vi "Logger.vi"(0 "Record":refnum<vi>, 1 "Indicators":T6, 2 "Time Stamp":refnum<vi>, 5 "Exit":refnum<vi>, 7 "Visual Data":T1, 9 "Period [ms]":i32=50, 11 "error in (no error)":errorcluster, 12 "File Path Control":refnum<vi>, 13 "Configuration":T5, 14 "Filename":string="RITA") -> (15 "error out":errorcluster)   [LabVIEW 2012, in "Logger VIs.lvlib"]
uses:
  Logger VIs.lvlib
  State.ctl
  <vilib>/silver_ctls/ArrayMatrixCluster/Real Matrix NI_Silver.ctl
  <vilib>/vision/Image Controls.llb/IMAQ Image.ctl
  <vilib>/Utility/xml.llb/Write to XML File(string).vi
panel:
  out "Transformation":T3
  out "Calibration":T4
  out "Angles":cluster{"Azimut":dbl, "Elevation":dbl}
  out "Surface Space":dbl
  out "ms from start":dbl
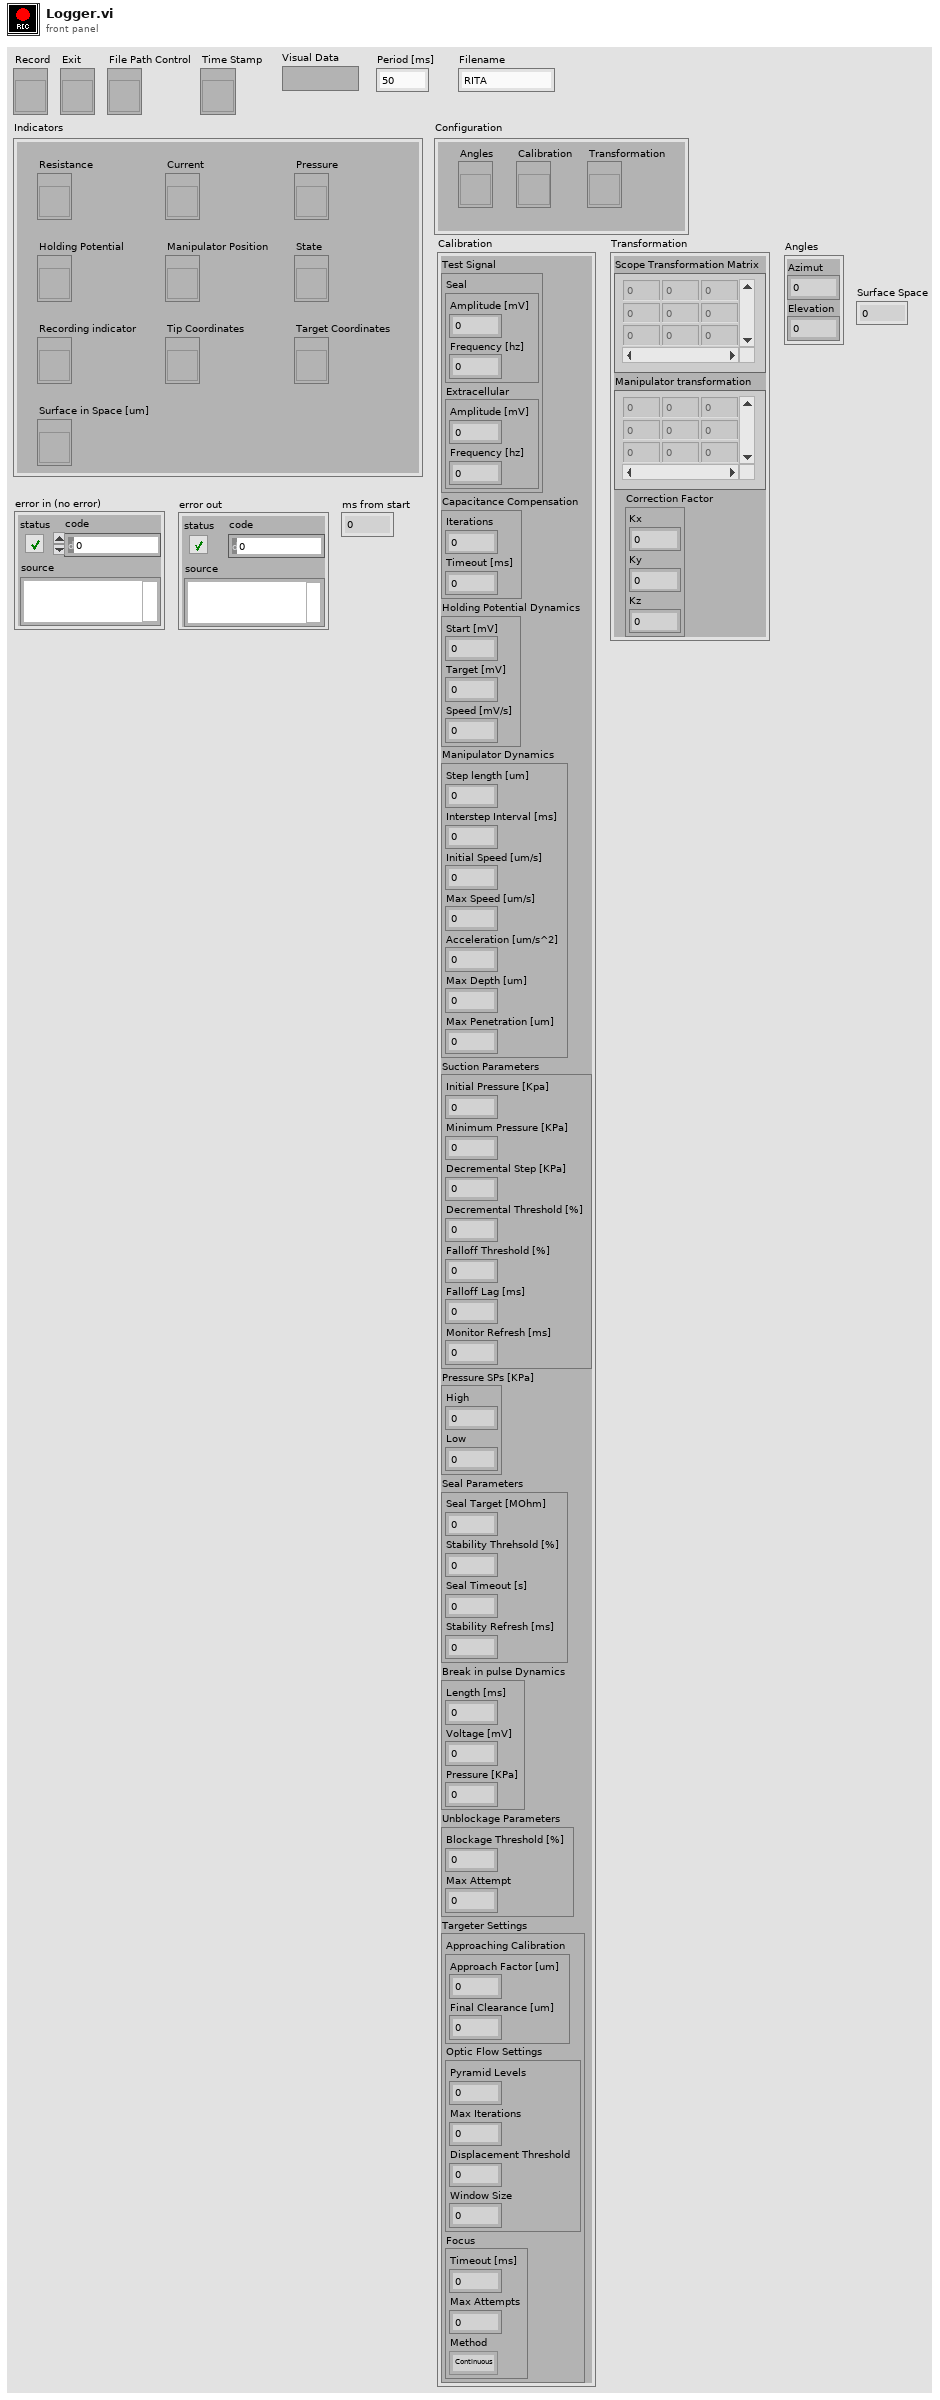
[diagram p1: front panel]
types:
  T1 = typedef "IMAQ Image.ctl" = refnum<image>
  T2 = typedef "Real Matrix NI_Silver.ctl" = dbl[][]
  T3 = cluster{"Scope Transformation Matrix":T2, "Manipulator transformation":T2, "Correction Factor":cluster{"Kx":dbl, "Ky":dbl, "Kz":dbl}}
  T4 = cluster{"Test Signal":cluster{"Seal":cluster{"Amplitude [mV]":i32, "Frequency [hz]":u16}, "Extracellular":cluster{"Amplitude [mV]":i32, "Frequency [hz]":u16}}, "Capacitance Compensation":cluster{"Iterations":i32, "Timeout [ms]":u32}, "Holding Potential Dynamics":cluster{"Start [mV]":dbl, "Target [mV]":dbl, "Speed [mV/s]":dbl}, "Manipulator Dynamics":cluster{"Step length [um]":dbl, "Interstep Interval [ms]":u32, "Initial Speed [um/s]":dbl, "Max Speed [um/s]":dbl, "Acceleration [um/s^2]":dbl, "Max Depth [um]":dbl, "Max Penetration [um]":dbl}, "Suction Parameters":cluster{"Initial Pressure [Kpa]":dbl, "Minimum Pressure [KPa]":dbl, "Decremental Step [KPa]":dbl, "Decremental Threshold [%]":dbl, "Falloff Threshold [%]":dbl, "Falloff Lag [ms]":dbl, "Monitor Refresh [ms]":dbl}, "Pressure SPs [KPa]":cluster{"High":dbl, "Low":dbl}, "Seal Parameters":cluster{"Seal Target [MOhm]":dbl, "Stability Threhsold [%]":dbl, "Seal Timeout [s]":dbl, "Stability Refresh [ms]":dbl}, "Break in pulse Dynamics":cluster{"Length [ms]":dbl, "Voltage [mV]":dbl, "Pressure [KPa]":dbl}, "Unblockage Parameters":cluster{"Blockage Threshold [%]":dbl, "Max Attempt":i32}, "Targeter Settings":cluster{"Approaching Calibration":cluster{"Approach Factor [um]":dbl, "Final Clearance [um]":dbl}, "Optic Flow Settings":cluster{"Pyramid Levels":i32, "Max Iterations":i32, "Displacement Threshold":dbl, "Window Size":i32}, "Focus":cluster{"Timeout [ms]":u32, "Max Attempts":u32, "Method":enum16{"Continuous", "On Demand"}}}}
  T5 = cluster{"Angles":refnum<vi>, "Calibration":refnum<vi>, "Transformation":refnum<vi>}
  T6 = cluster{"Current":refnum<vi>, "Holding Potential":refnum<vi>, "Recording indicator":refnum<vi>, "Pressure":refnum<vi>, "Resistance":refnum<vi>, "Manipulator Position":refnum<vi>, "Tip Coordinates":refnum<vi>, "Target Coordinates":refnum<vi>, "Surface in Space [um]":refnum<vi>, "State":refnum<vi>}
  T7 = enum16{"open", "replace", "create", "open or create", "replace or create", "replace or create with confirmation"}
  T8 = cluster{"Value":dbl, "Value 2":dbl, "Value 3":dbl}
  T9 = cluster{"X [um]":dbl, "Y [um]":dbl, "Z [um]":dbl}
  T10 = typedef "State.ctl" = enum16{"READY", "LOAD", "LOCALIZATION", "HUNTING", "SEAL", "BREAKIN", "WCR", "ALIGN", "APPROACH", "TARGETING"}
  T11 = cluster{"Scope Transformation Matrix":T2, "Manipulator transformation":T2, "Coorection Factor":cluster{"Kx":dbl, "Ky":dbl, "Kz":dbl}}
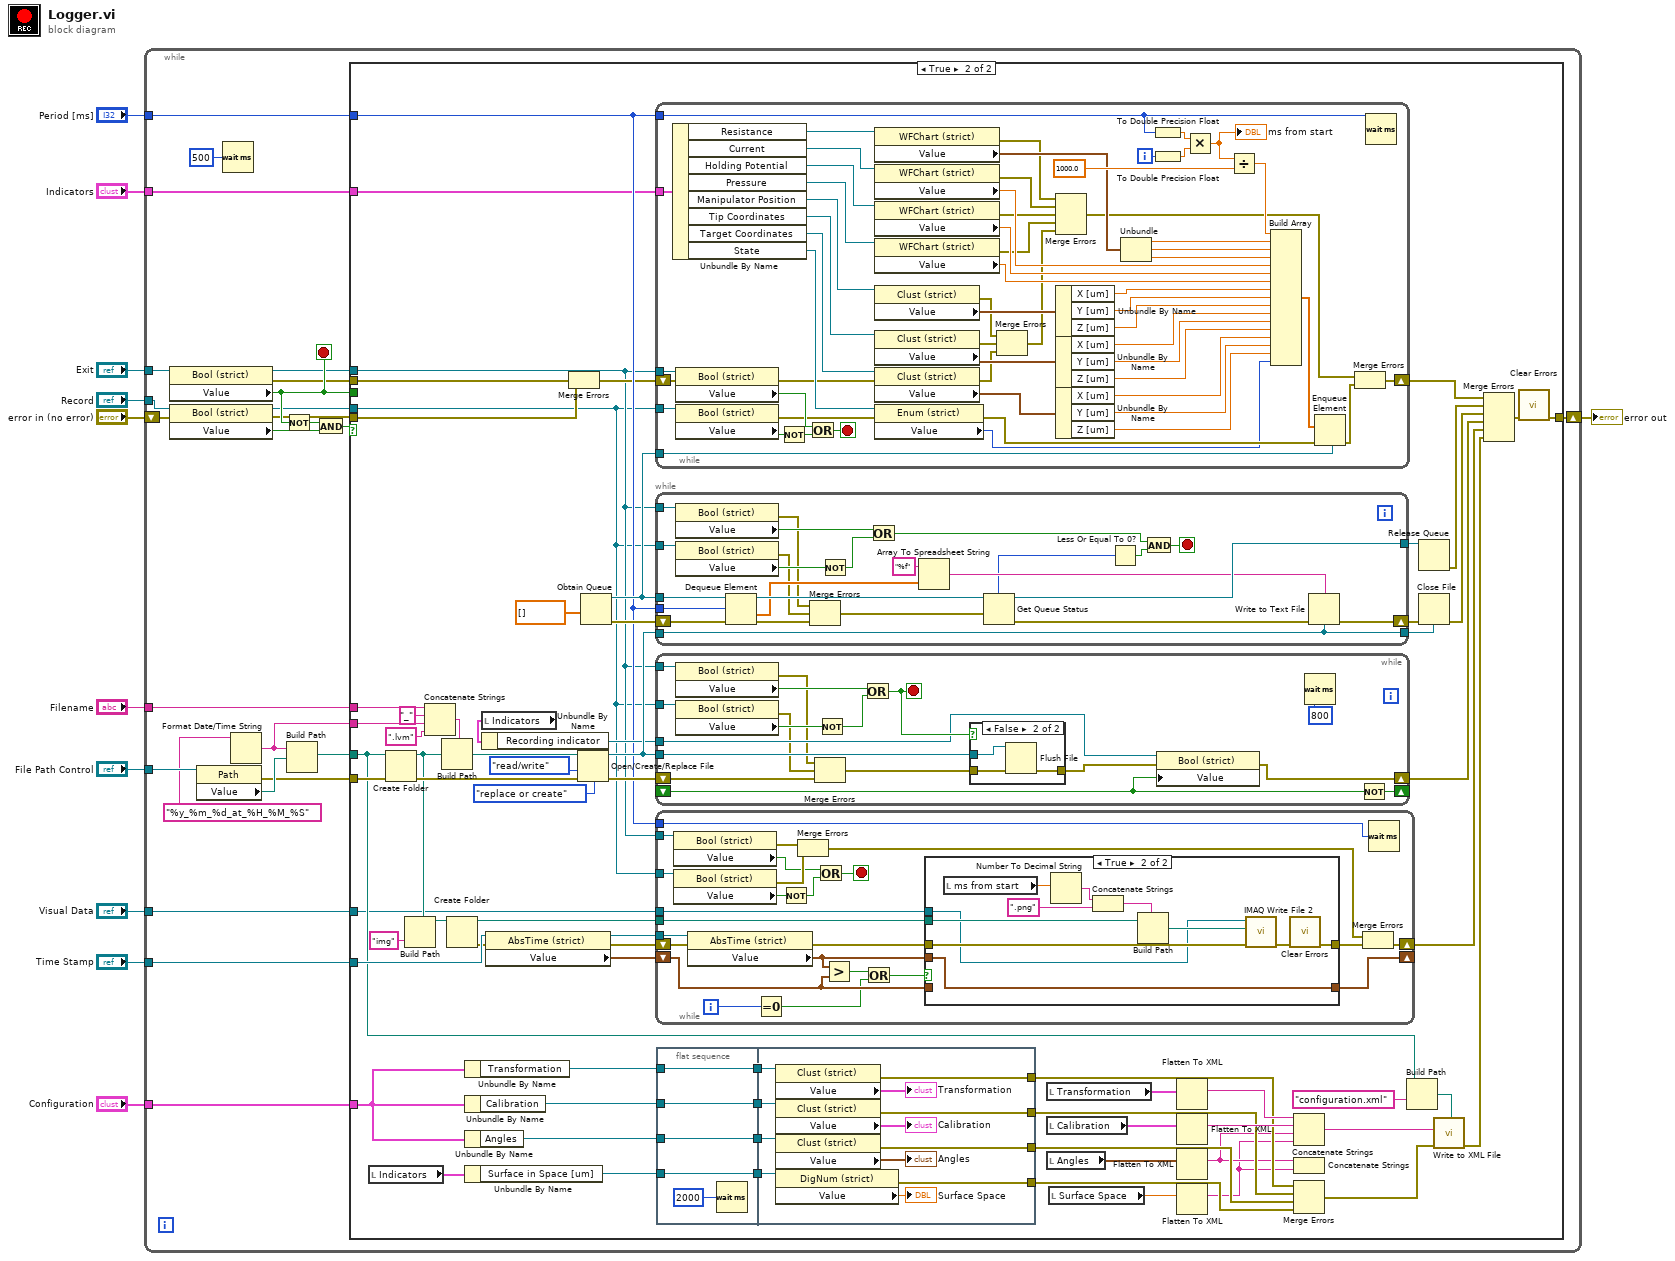
[diagram p0: block diagram]
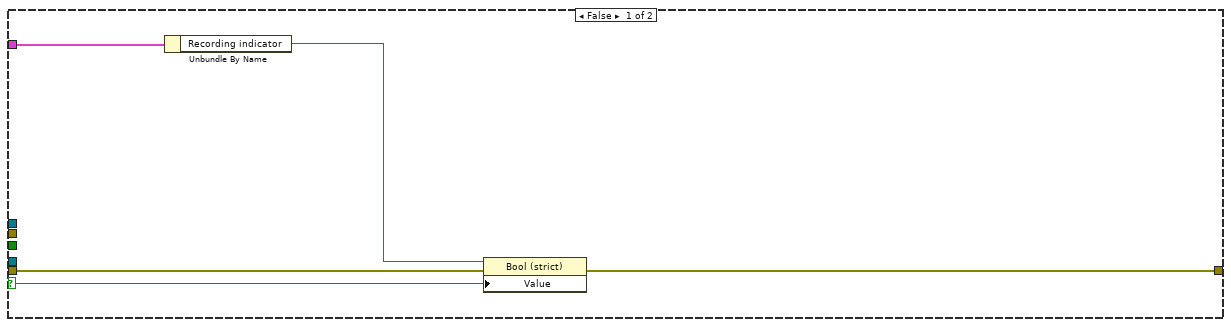
[diagram p2: hidden frame]
diagram:
  n1 = while {
    tunnel: "Indicators" -> [w35]
    tunnel: "Period [ms]" -> [w36]
    tunnel: "Exit" -> [w16]
    tunnel: "Record" -> [w17]
    shift-right: [w31] -> w7
    shift-left: "error in (no error)" -> [w13]
    tunnel: "File Path Control" -> [w32]
    tunnel: "Filename" -> [w30]
    tunnel: "Time Stamp" -> [w15]
    tunnel: "Configuration" -> [w14]
    tunnel: "Visual Data" -> [w12]
    stop <- w33 stop-if-true
    n2 = property class="Bool (strict)"(reference=w16) -> (reference out=w28:refnum<vi>, error out=w20:errorcluster, "Value"=w33:bool)  [unwired: 1 in]
    n3 = property class="Bool (strict)"(reference=w17, error in=w13) -> (reference out=w29:refnum<vi>, error out=w19:errorcluster, "Value"=w26:bool)
    n4 = property class="Path"(reference=w32) -> (error out=w21:errorcluster, "Value"=w24:path)  [unwired: 1 in, 1 out]
    n5 = Wait (ms)(milliseconds to wait=u32 500) -> ()  [unwired: 1 out]
    n6 = Format Date/Time String(time format string (%c)="%y_%m_%d_at_%H_%M_%S") -> (date/time string=w22:string)  [unwired: 2 in]
    n7 = Not(x=w33) -> (.not. x?=w25:bool)
    n8 = Build Path(base path=w24, name or relative path=w22) -> (appended path=w23:path)
    n9 = And(x=w25, y=w26) -> (x .and. y?=w27:bool)
    n10 = case shown="True" w27 {
      selector: w27 -> [w39 _]
      tunnel: w35 -> [w41 w79]
      tunnel: w36 -> [_ w80]
      tunnel: w29 -> [_ w48]
      tunnel: w33 -> [_ _]
      tunnel: w28 -> [_ w49]
      tunnel: [w38 w44] -> w31
      tunnel: w23 -> [_ w71]
      tunnel: w22 -> [_ w96]
      tunnel: w30 -> [_ w90]
      tunnel: w21 -> [_ w92]
      tunnel: w20 -> [_ w51]
      tunnel: w19 -> [w37 w50]
      tunnel: w15 -> [_ w85]
      tunnel: w14 -> [_ w73]
      tunnel: w12 -> [_ w46]
      frame False {
        n11 = Unbundle By Name(w41) -> ("Recording indicator"=w40:refnum<vi>)
        n12 = property class="Bool (strict)"(reference=w40, error in=w37, "Value"=w39) -> (error out=w38:errorcluster)  [unwired: 1 out]
      }
      frame True {
        n13 = local read "Indicators"() -> (w69:T6)
        n14 = Create Folder(path (use dialog)=w71, error in=w92) -> (created path=w93:path, error out=w94:errorcluster)  [unwired: 1 in, 1 out]
        n15 = Build Path(base path=w93, name or relative path="img") -> (appended path=w88:path)
        n16 = Concatenate Strings(w90, "_" ("string"), w96, ".lvm" ("time format string (%c)")) -> (w97:string)
        n17 = Build Path(base path=w93, name or relative path=w97) -> (appended path=w95:path)
        n18 = Create Folder(path (use dialog)=w88) -> (created path=w86:path, error out=w84:errorcluster)  [unwired: 2 in, 1 out]
        n19 = Unbundle By Name(w73) -> ("Transformation"=w76:refnum<vi>)
        n20 = Unbundle By Name(w73) -> ("Calibration"=w74:refnum<vi>)
        n21 = Unbundle By Name(w73) -> ("Angles"=w72:refnum<vi>)
        n22 = Unbundle By Name(w69) -> ("Surface in Space [um]"=w43:refnum<vi>)
        n23 = local read "Indicators"() -> (w75:T6)
        n24 = Unbundle By Name(w75) -> ("Recording indicator"=w103:refnum<vi>)
        n25 = property class="AbsTime (strict)"(reference=w85, error in=w84) -> (reference out=w81:refnum<vi>, error out=w82:errorcluster, "Value"=w83:timestamp)
        n26 = Merge Errors(w51, w50) -> (w52:errorcluster)
        n27 = Open/Create/Replace File(file path (use dialog)=w95, error in=w94, operation (0:open)=T7."replace or create", access (0:read/write)=enum16{"read/write", "read-only", "write-only"}."read/write") -> (refnum out=w107:refnum<file>, error out=w108:errorcluster)  [unwired: 2 in, 1 out]
        n28 = Obtain Queue(element data type=dbl[] [] ("array")) -> (queue out=w109:refnum<queue>, error out=w105:errorcluster)  [unwired: 4 in, 1 out]
        n29 = while {
          tunnel: w109 -> [w226]
          tunnel: w79 -> [w223]
          tunnel: w49 -> [w207]
          tunnel: w48 -> [w206]
          tunnel: w80 -> [w198]
          shift-right: [w180] -> w102
          shift-left: w52 -> [w168]
          i -> [w199]
          stop <- w205 stop-if-true
          n30 = Unbundle By Name(w223) -> ("Resistance"=w222:refnum<vi>, "Current"=w221:refnum<vi>, "Holding Potential"=w219:refnum<vi>, "Pressure"=w216:refnum<vi>, "Manipulator Position"=w215:refnum<vi>, "Tip Coordinates"=w194:refnum<vi>, "Target Coordinates"=w193:refnum<vi>, "State"=w196:refnum<vi>)
          n31 = property class="Bool (strict)"(reference=w207, error in=w168) -> (error out=w191:errorcluster, "Value"=w208:bool)  [unwired: 1 out]
          n32 = property class="Bool (strict)"(reference=w206) -> (error out=w190:errorcluster, "Value"=w209:bool)  [unwired: 1 in, 1 out]
          n33 = Not(x=w209) -> (.not. x?=w210:bool)
          n34 = Or(x=w208, y=w210) -> (x .or. y?=w205:bool)
          n35 = property class="WFChart (strict)"(reference=w222) -> (error out=w185:errorcluster, "Value"=w203:T8)  [unwired: 1 in, 1 out]
          n36 = property class="WFChart (strict)"(reference=w221) -> (error out=w186:errorcluster, "Value"=w220:dbl)  [unwired: 1 in, 1 out]
          n37 = property class="WFChart (strict)"(reference=w219) -> (error out=w187:errorcluster, "Value"=w218:dbl)  [unwired: 1 in, 1 out]
          n38 = property class="WFChart (strict)"(reference=w216) -> (error out=w188:errorcluster, "Value"=w217:dbl)  [unwired: 1 in, 1 out]
          n39 = property class="Clust (strict)"(reference=w215) -> (error out=w182:errorcluster, "Value"=w214:T9)  [unwired: 1 in, 1 out]
          n40 = property class="Clust (strict)"(reference=w194) -> (error out=w183:errorcluster, "Value"=w195:T9)  [unwired: 1 in, 1 out]
          n41 = property class="Clust (strict)"(reference=w193, error in=w191) -> (error out=w184:errorcluster, "Value"=w192:T9)  [unwired: 1 out]
          n42 = property class="Enum (strict)"(reference=w196, error in=w190) -> (error out=w189:errorcluster, "Value"=w177:T10)  [unwired: 1 out]
          n43 = Merge Errors(w182, w183, w184) -> (w181:errorcluster)
          n44 = Merge Errors(w185, w186, w187, w188, w181) -> (w179:errorcluster)
          n45 = Unbundle By Name(w214) -> ("X [um]"=w213:dbl, "Y [um]"=w212:dbl, "Z [um]"=w211:dbl)
          n46 = Unbundle By Name(w195) -> ("X [um]"=w174:dbl, "Y [um]"=w173:dbl, "Z [um]"=w172:dbl)
          n47 = Unbundle By Name(w192) -> ("X [um]"=w171:dbl, "Y [um]"=w170:dbl, "Z [um]"=w169:dbl)
          n48 = Unbundle(w203) -> ("Value"=w202:dbl, "Value 2"=w201:dbl, "Value 3"=w200:dbl)
          n49 = To Double Precision Float(number=w198) -> (double precision float=w176:dbl)
          n50 = To Double Precision Float(number=w199) -> (double precision float=w175:dbl)
          n51 = Multiply(x=w176, y=w175) -> (x*y=w197:dbl)
          "ms from start" <- w197
          n52 = Divide(x=w197, y=1000.0) -> (x/y=w204:dbl)
          n53 = Build Array(w204, w202, w201, w200, w220, w218, w217, w213, w212, w211, w174, w173, w172, w171, w170, w169, w177) -> (w224:dbl[])
          n54 = Enqueue Element(queue=w226, element=w224, error in (no error)=w189) -> (error out=w178:errorcluster)  [unwired: 1 in, 2 out]
          n55 = Merge Errors(w179, w178) -> (w180:errorcluster)
          n56 = Wait (ms)(milliseconds to wait=w198) -> ()  [unwired: 1 out]
        }
        n57 = while {
          tunnel: [w249] -> w113
          tunnel: w109 -> [w248]
          tunnel: w49 -> [w246]
          tunnel: w48 -> [w245]
          tunnel: w107 -> [w236]
          tunnel: [w236] -> w106
          tunnel: w80 -> [w231]
          shift-right: [w247] -> w104
          shift-left: w105 -> [w232]
          stop <- w237 stop-if-true
          n58 = property class="Bool (strict)"(reference=w246) -> (error out=w228:errorcluster, "Value"=w240:bool)  [unwired: 1 in, 1 out]
          n59 = property class="Bool (strict)"(reference=w245) -> (error out=w229:errorcluster, "Value"=w239:bool)  [unwired: 1 in, 1 out]
          n60 = Dequeue Element(queue=w248, timeout in ms (-1)=w231, error in (no error)=w232) -> (element=w243:dbl[], error out=w230:errorcluster)  [unwired: 2 out]
          n61 = Merge Errors(w228, w229, w230) -> (w227:errorcluster)
          n62 = Not(x=w239) -> (.not. x?=w241:bool)
          n63 = Or(x=w240, y=w241) -> (x .or. y?=w238:bool)
          n64 = Array To Spreadsheet String(array=w243, 3:"%f" ("format string")) -> (spreadsheet string=w244:string)  [unwired: 1 out]
          n65 = Get Queue Status(queue=w248, error in (no error)=w227) -> (queue out=w249:refnum<queue>, error out=w242:errorcluster, # elements in queue=w234:i32)  [unwired: 6 out]
          n66 = Less Or Equal To 0?(x=w234) -> (x <= 0?=w233:bool)
          n67 = And(x=w238, y=w233) -> (x .and. y?=w237:bool)
          n68 = Write to Text File(file (use dialog)=w236, text=w244, error in=w242) -> (error out=w247:errorcluster)  [unwired: 1 in, 2 out]
        }
        n69 = while {
          tunnel: w107 -> [w266]
          tunnel: w49 -> [w264]
          tunnel: w48 -> [w263]
          shift-right: [w256] -> w99
          shift-left: w108 -> [w251]
          shift-right: [w259] -> _
          shift-left: _ -> [w258]
          tunnel: w103 -> [w254]
          stop <- w257 stop-if-true
          n70 = property class="Bool (strict)"(reference=w264) -> (error out=w253:errorcluster, "Value"=w261:bool)  [unwired: 1 in, 1 out]
          n71 = property class="Bool (strict)"(reference=w263) -> (error out=w252:errorcluster, "Value"=w262:bool)  [unwired: 1 in, 1 out]
          n72 = Merge Errors(w253, w252, w251) -> (w250:errorcluster)
          n73 = Not(x=w262) -> (.not. x?=w260:bool)
          n74 = Or(x=w261, y=w260) -> (x .or. y?=w257:bool)
          n75 = case shown="False" w257 {
            tunnel: w266 -> [_ w270]
            tunnel: w250 -> [w267 w269]
            tunnel: [w267 w268] -> w255
            frame True {
            }
            frame False {
              n76 = Flush File(refnum=w270, error in=w269) -> (error out=w268:errorcluster)  [unwired: 1 out]
            }
          }
          n77 = property class="Bool (strict)"(reference=w254, error in=w255, "Value"=w258) -> (error out=w256:errorcluster)  [unwired: 1 out]
          n78 = Wait (ms)(milliseconds to wait=u32 800) -> ()  [unwired: 1 out]
          n79 = Not(x=w258) -> (.not. x?=w259:bool)
        }
        n80 = while {
          tunnel: w86 -> [w154]
          shift-right: [w139] -> w98
          shift-left: w82 -> [w147]
          shift-right: [w143] -> _
          shift-left: w83 -> [w144]
          tunnel: w81 -> [w148]
          tunnel: w49 -> [w142]
          tunnel: w48 -> [w141]
          tunnel: w80 -> [w136]
          tunnel: w46 -> [w135]
          i -> [w134]
          stop <- w151 stop-if-true
          n81 = property class="Bool (strict)"(reference=w142) -> (error out=w149:errorcluster, "Value"=w137:bool)  [unwired: 1 in, 1 out]
          n82 = property class="Bool (strict)"(reference=w141) -> (error out=w150:errorcluster, "Value"=w153:bool)  [unwired: 1 in, 1 out]
          n83 = property class="AbsTime (strict)"(reference=w148, error in=w147) -> (error out=w146:errorcluster, "Value"=w145:timestamp)  [unwired: 1 out]
          n84 = Equal To 0?(x=w134) -> (x = 0?=w131:bool)
          n85 = Not(x=w153) -> (.not. x?=w152:bool)
          n86 = Merge Errors(w149, w150) -> (w138:errorcluster)
          n87 = Or(x=w137, y=w152) -> (x .or. y?=w151:bool)
          n88 = Greater?(x=w145, y=w144) -> (0:w132:bool)
          n89 = Or(x=w132, y=w131) -> (x .or. y?=w133:bool)
          n90 = case shown="True" w133 {
            tunnel: w154 -> [_ w160]
            tunnel: [w156 w157] -> w140
            tunnel: w146 -> [w156 w161]
            tunnel: w145 -> [_ w163]
            tunnel: w144 -> [w155 _]
            tunnel: [w155 w163] -> w143
            tunnel: w135 -> [_ w159]
            frame False {
            }
            frame True {
              n91 = local read "ms from start"() -> (w164:dbl)
              n92 = Number To Decimal String(number=w164) -> (decimal integer string=w167:string)  [unwired: 1 in]
              n93 = Concatenate Strings(w167, ".png" ("string")) -> (w165:string)
              n94 = Build Path(base path=w160, name or relative path=w165) -> (appended path=w162:path)
              n95 = call-poly "IMAQ Write File 2"("error in (no error)"=w161, "File Path"=w162, "Image"=w159) -> ("error out"=w158:errorcluster)  [unwired: 7 in, 1 out]
              n96 = call <vilib>:"Clear Errors.vi"("error in (no error)"=w158) -> ("error out"=w157:errorcluster)  [unwired: 6 in]
            }
          }
          n97 = Merge Errors(w138, w140) -> (w139:errorcluster)
          n98 = Wait (ms)(milliseconds to wait=w136) -> ()  [unwired: 1 out]
        }
        n99 = flat-sequence {
          tunnel: w43 -> [w115]
          tunnel: w72 -> [w116]
          tunnel: w74 -> [w117]
          tunnel: w76 -> [w118]
          tunnel: [w118] -> w56
          tunnel: [w117] -> w55
          tunnel: [w116] -> w54
          tunnel: [w115] -> w53
          tunnel: [w126] -> w68
          tunnel: [w125] -> w67
          tunnel: [w124] -> w66
          tunnel: [w123] -> w65
          tunnel: w56 -> [w130]
          tunnel: w55 -> [w129]
          tunnel: w54 -> [w128]
          tunnel: w53 -> [w127]
          frame #0 {
            n100 = Wait (ms)(milliseconds to wait=u32 2000) -> ()  [unwired: 1 out]
          }
          frame #1 {
            n101 = property on="Property Node" class="Clust (strict)"(reference=w130) -> (error out=w126:errorcluster, "Value"=→"Transformation":T11)  [unwired: 1 in, 1 out]
            n102 = property on="Property Node" class="Clust (strict)"(reference=w129) -> (error out=w125:errorcluster, "Value"=→"Calibration":T4)  [unwired: 1 in, 1 out]
            n103 = property on="Property Node" class="Clust (strict)"(reference=w128) -> (error out=w124:errorcluster, "Value"=→"Angles":cluster{"Azimut":dbl, "Elevation":dbl})  [unwired: 1 in, 1 out]
            n104 = property on="Property Node" class="DigNum (strict)"(reference=w127) -> (error out=w123:errorcluster, "Value"=→"Surface Space":dbl)  [unwired: 1 in, 1 out]
          }
        }
        n105 = local read "Transformation"() -> (w60:T3)
        n106 = local read "Calibration"() -> (w61:T4)
        n107 = local read "Angles"() -> (w62:cluster{"Azimut":dbl, "Elevation":dbl})
        n108 = local read "Surface Space"() -> (w63:dbl)
        n109 = Flatten To XML(anything=w60) -> (xml string=w78:string)
        n110 = Flatten To XML(anything=w61) -> (xml string=w77:string)
        n111 = Flatten To XML(anything=w62) -> (xml string=w59:string)
        n112 = Flatten To XML(anything=w63) -> (xml string=w58:string)
        n113 = Concatenate Strings(w78, w77, w59, w58) -> (w57:string)
        n114 = Concatenate Strings(w59, w58) -> ()  [unwired: 1 out]
        n115 = Merge Errors(w68, w67, w66, w65) -> (w64:errorcluster)
        n116 = Build Path(base path=w71, name or relative path="configuration.xml") -> (appended path=w42:path)
        n117 = Release Queue(queue=w113) -> (error out=w101:errorcluster)  [unwired: 1 in, 3 out]
        n118 = Close File(refnum=w106, error in=w104) -> (error out=w100:errorcluster)  [unwired: 1 out]
        n119 = call-poly <vilib>:"Write to XML File.vi"("error in (no error)"=w64, "XML Input"=w57, "XML File Path"=w42) -> ("error out"=w47:errorcluster)  [unwired: 2 in, 6 out]
        n120 = Merge Errors(w102, w101, w100, w99, w98, w47) -> (w45:errorcluster)
        n121 = call <vilib>:"Clear Errors.vi"("error in (no error)"=w45) -> ("error out"=w44:errorcluster)  [unwired: 6 in]
      }
    }
  }
  "error out" <- w7
